vi "ExSub5CalGlueLive1NI.vi"(2 "Lower limit":dbl format="%.2f", 3 "Upper limit":dbl format="%.2f", 4 "error in (no error)":errorcluster, 5 "String":string, 6 "Resolution":dbl format="%.2f", 7 "Image Handle":u32) -> (0 "error out":errorcluster, 1 "Glue handle":u32)   [LabVIEW 2010]
panel:
  # "ExSub5CalGlueLIve1NI.vi : this sub vi takes a frame of 5 \nstrips and glues it using special calibration ini file."
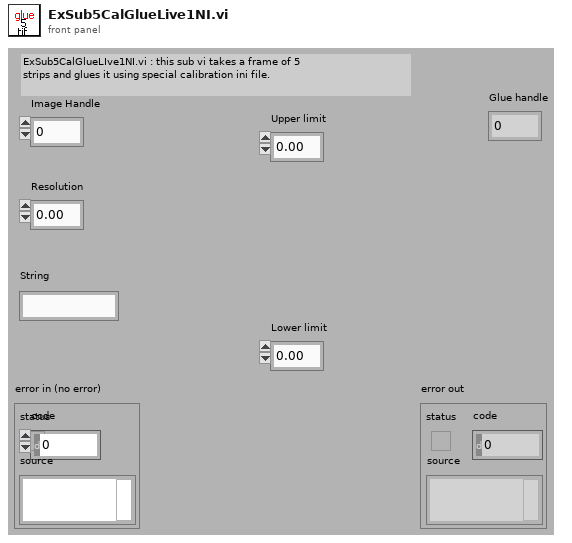
[diagram p1: front panel]
types:
  T1 = cluster{"Upper limit":dbl, "Lower limit":dbl, "Resolution":dbl, "wavelenght":i32}
  T2 = cluster{"Pixel width\nmicrons":i32, "Pixel width\nmicrons":i32, i32, "Y dim":i32, i32}
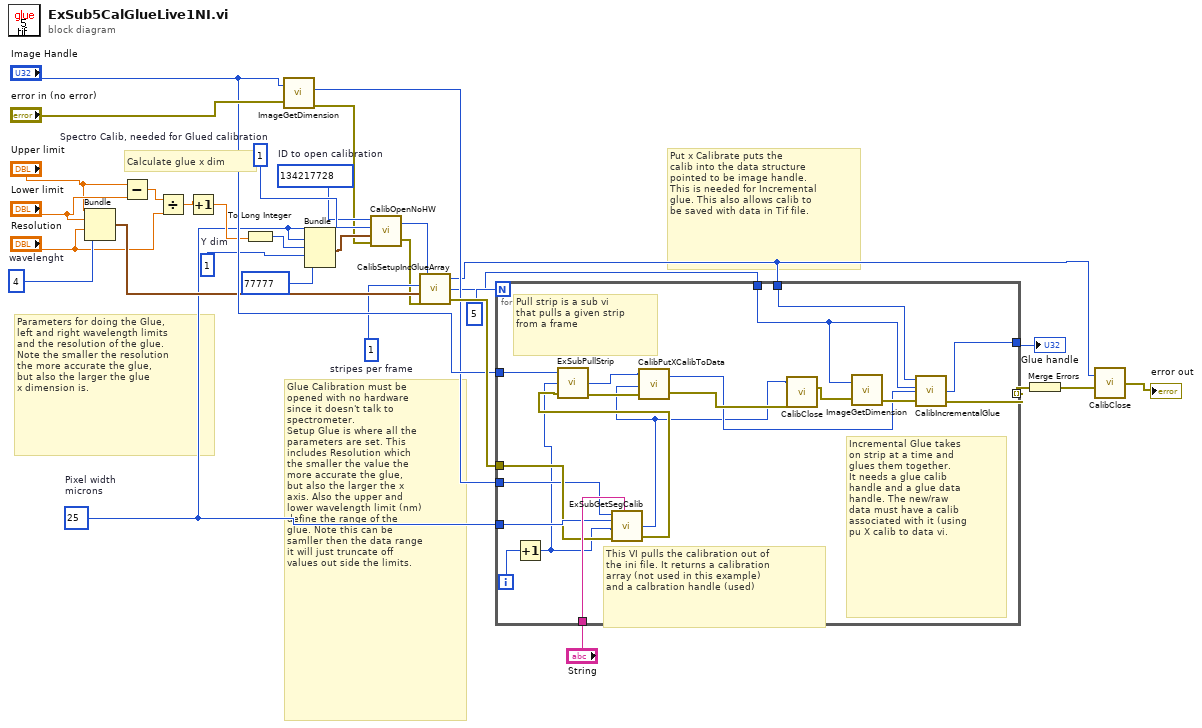
[diagram p0: block diagram]
diagram:
  w18 = 1  # stripes per frame
  w20 = 4  # wavelenght
  w4 = 25  # Pixel width microns
  w13 = 1  # Y dim
  w28 = 1  # Spectro Calib, needed for Glued calibration
  w27 = 134217728  # ID to open calibration
  # "Put x Calibrate puts the\ncalib into the data structure \npointed to be image handle. \nThis is needed for Incremental\nglue. This also allows calib to\nbe saved with data in Tif file."
  # "Glue Calibration must be \nopened with no hardware\nsince it doesn't talk to \nspectrometer.\nSetup Glue is where all the\nparameters are set. This\nincludes Resolution which\nthe smaller the value the \nmore accurate the glue, \nbut also the larger the x\naxis. Also the upper and\nlower wavelength limit (nm)\ndefine the range of the \nglue. Note this can be \nsamller then the data range\nit will just truncate off \nvalues out side the limits."
  # "Parameters for doing the Glue,\nleft and right wavelength limits \nand the resolution of the glue.\nNote the smaller the resolution \nthe more accurate the glue, \nbut also the larger the glue\nx dimension is."
  # "Calculate glue x dim"
  n1 = Bundle("Upper limit"="Upper limit", "Lower limit"="Lower limit", "Resolution"="Resolution", "wavelenght"=w20) -> (w19:T1)  [unwired: 1 in]
  n2 = Subtract(x="Upper limit", y="Lower limit") -> (x-y=w16:dbl)
  n3 = Divide(x=w16, y="Resolution") -> (x/y=w15:dbl)
  n4 = Increment(x=w15) -> (x+1=w12:dbl)
  n5 = To Long Integer(number=w12) -> (32bit integer=w14:i32)
  n6 = call <userlib>:"ImageGetDimension.vi"("Image Handle"="Image Handle", "error in"="error in (no error)") -> ("X dimension"=w17:u32, "error out"=w24:errorcluster)  [unwired: 4 out]
  n7 = Bundle("Pixel width\nmicrons"=w4, "Pixel width\nmicrons"=w4, w14, "Y dim"=w13, 77777) -> (w29:T2)  [unwired: 1 in]
  n8 = call <userlib>:"CalibOpenNoHW.vi"("error in"=w24, "Data Info"=w29, "Calibration Type"=w28, "Calibration Device ID"=w27) -> ("error out"=w5:errorcluster, "Calibration Handle"=w26:u32)
  n9 = call <userlib>:"CalibSetupIncGlueArray.vi"("error in (no error)"=w5, "Glue Output Params"=w19, "StripsPerFrame"=w18, "Calibration Handle"=w26) -> ("error out"=w23:errorcluster, "Glued Data Handle"=w11:u32, "Calibration Handle"=w10:u32)
  n10 = for {
    N: 5 -> [_]
    tunnel: "String" -> [w50]
    tunnel: w17 -> [w42]
    tunnel: w4 -> [w49]
    tunnel: w23 -> [w47]
    tunnel: "Image Handle" -> [w43]
    tunnel: w11 -> [w39]
    tunnel: w10 -> [w40]
    tunnel: [w37] -> w3
    tunnel: [w32] -> w2 mode=indexing
    i -> [w48]
    # "Incremental Glue takes\non strip at a time and \nglues them together.\nIt needs a glue calib\nhandle and a glue data \nhandle. The new/raw \ndata must have a calib\nassociated with it (using\npu X calib to data vi."
    # "Pull strip is a sub vi\nthat pulls a given strip\nfrom a frame"
    # "This VI pulls the calibration out of\nthe ini file. It returns a calibration\narray (not used in this example) \nand a calbration handle (used)"
    n11 = Increment(x=w48) -> (x+1=w41:i32)
    n12 = call "ExSubGetSegCalib.vi"("x dimension"=w42, "Pixel width"=w49, "Segment number"=w41, "error in (no error)"=w47, "ini file"=w50) -> ("Calibration Handle"=w33:u32, "error out"=w46:errorcluster)  [unwired: 1 out]
    n13 = call "ExSubPullStrip.vi"("error in (no error)"=w46, "Strip to pull out"=w41, "Image Handle"=w43) -> ("error out"=w45:errorcluster, "New Image Handle"=w44:u32)  [unwired: 1 out]
    n14 = call <userlib>:"CalibPutXCalibToData.vi"("error in (no error)"=w45, "Calibration Handle"=w33, "Data Handle"=w44) -> ("error out"=w36:errorcluster, "Data Handle"=w34:u32)
    n15 = call <userlib>:"CalibClose.vi"("error in"=w36, "Calibration Handle"=w33) -> ("error out"=w35:errorcluster)
    n16 = call <userlib>:"ImageGetDimension.vi"("Image Handle"=w39, "error in"=w35) -> ("error out"=w38:errorcluster)  [unwired: 5 out]
    n17 = call <userlib>:"CalibIncrementalGlue.vi"("error in (no error)"=w38, "Raw Data Handle"=w34, "Result Data Handle"=w39, "Calibration Handle"=w40) -> ("error out"=w32:errorcluster, "Result Data Handle"=w37:u32)  [unwired: 1 out]
  }
  "Glue handle" <- w3
  n18 = Merge Errors(w2) -> (w9:errorcluster)
  n19 = call <userlib>:"CalibClose.vi"("error in"=w9, "Calibration Handle"=w10) -> ("error out"=→"error out":errorcluster)
